vi "MPZ2006固态源.vi"() -> ()   [LabVIEW 2015]
doc: "使用该模板构建用户界面事件处理设计模式。将模板应用于对话框及其它用户界面。用户也可创建并执行VI可按照与用户界面事件相同方式处理的用户定义事件。"
uses:
  <vilib>/Instr/_visa.llb/VISA Configure Serial Port (Instr).vi
panel:
  in  "预备区功率":string
  in  "写入功率控制表":bool caption="按钮1"
  in  "写标定功率检测值":bool caption="按钮1"
  in  "标定参数表":string[][](table)=[["034B", "0412", "04D8", "059F", "0666"], ["149B", "1735", "1A3D", "1D43", "2CCC"], ["15C2", "17AD", "1AE1", "1DE6", "30A3"], ["2851", "2851", "2851", "2851", "2851"], ["2D70", "2D70", "2D70", "2D70", "2D70"]]
  out "功率输出状态":bool
  in  "功率输出":bool
  in  "自动计算参数":bool caption="按钮1"
  in  "读标定功率检测值":bool caption="按钮1"
  in  "偏置2设置 2":dbl max=16383.0 format="%.4f"
  in  "偏置1设置 2":dbl max=16383.0 format="%.4f"
  in  "衰减器2设置 2":dbl max=16383.0 format="%.4f"
  in  "衰减器1设置 2":dbl max=16383.0 format="%.4f"
  out "状态数据":string[](array[string])
  out "串口":bool
  in  "驻波比limit设置":u16=10 min=10 max=99 format="%.0x"
  out "驻波比limit计算":string
  out "驻波比":string
  in  "开始上传":bool caption="按钮1"
  in  "开始下载":bool caption="按钮1"
  out "进度":u8(slide) scale=0.0..100.0
  in  "清空缓冲区":bool caption="按钮1"
  in  "导入模板文件":bool caption="按钮1"
  in  "保存文件":bool caption="按钮1"
  in  "功率控制表":string[][](table)
  in  "偏置2":u16 max=16383 format="%.0x"
  in  "偏置1":u16 max=16383 format="%.0x"
  in  "衰减器2":u16 max=16383 format="%.0x"
  in  "衰减器1":u16 max=16383 format="%.0x"
  in  "复制到数据缓冲区-->":bool caption="按钮1"
  in  "<--复制到控制窗":bool caption="按钮1"
  in  "备注":string
  out "温度limit计算":string
  out "电流limit计算":string
  in  "偏置2设置":u16 max=16383 format="%.0x"
  in  "偏置1设置":u16 max=16383 format="%.0x"
  in  "衰减器2设置":u16 max=16383 format="%.0x"
  in  "衰减器1设置":u16 max=16383 format="%.0x"
  in  "反向功率limit设置":u16 max=4095 format="%.0x"
  in  "正向功率limit设置":u16 max=4095 format="%.0x"
  in  "温度limit设置":u16 max=4095 format="%.0x"
  in  "电流limit设置":u16 max=4095 format="%.0x"
  in  "频率设置":dbl format="%#_6f"
  out "偏置2计算":string
  out "偏置1计算":string
  out "衰减器2计算":string
  out "衰减器1计算":string
  out "反向功率limit计算":string
  out "正向功率limit计算":string
  in  "设置参数":bool caption="按钮1"
  in  "保存数据":bool caption="按钮1"
  out "功率状态":enum16{"OFF", "ON"}(ring)
  out "偏置2 (V)":string
  out "偏置1 (V)":string
  out "衰减器2 (V)":string
  out "衰减器1 (V)":string
  out "驻波比limit":string
  out "反向功率limit (V/W/dBm)":string
  out "正向功率limit (V/W/dBm)":string
  out "温度limit (℃)":string
  out "电流limit（A）":string
  out "反向功率(V/W/dBm)":string
  out "正向功率(V/W/dBm)":string
  out "温度（℃）":string
  out "电流（A）":string
  out "频率（Hz）":string
  out "报警状态":string
  out "功率输出状态":string
  out "SN":string
  out "型号":string
  out "接收的原始数据":string
  in  "波特率":u32(ring)=19200 items=["75"=75, "110"=110, "134"=134, "150"=150, "300"=300, "600"=600, "1200"=1200, "1800"=1800, "2400"=2400, "4800"=4800, "7200"=7200, "9600"=9600, "14400"=14400, "19200"=19200, "28800"=28800, "38400"=38400, "56000"=56000, "57600"=57600, "115200"=115200, "128000"=128000, "230400"=230400]
  in  "串口号":refnum<visa-resource-name>="COM1"
  in  "打开串口":bool caption="按钮1"
  in  "stop":bool caption="停止"
  # "A"
  # "预备区"
  # "℃"
  # "W"
  # "W"
  # "V"
  # "V"
  # "V"
  # "V"
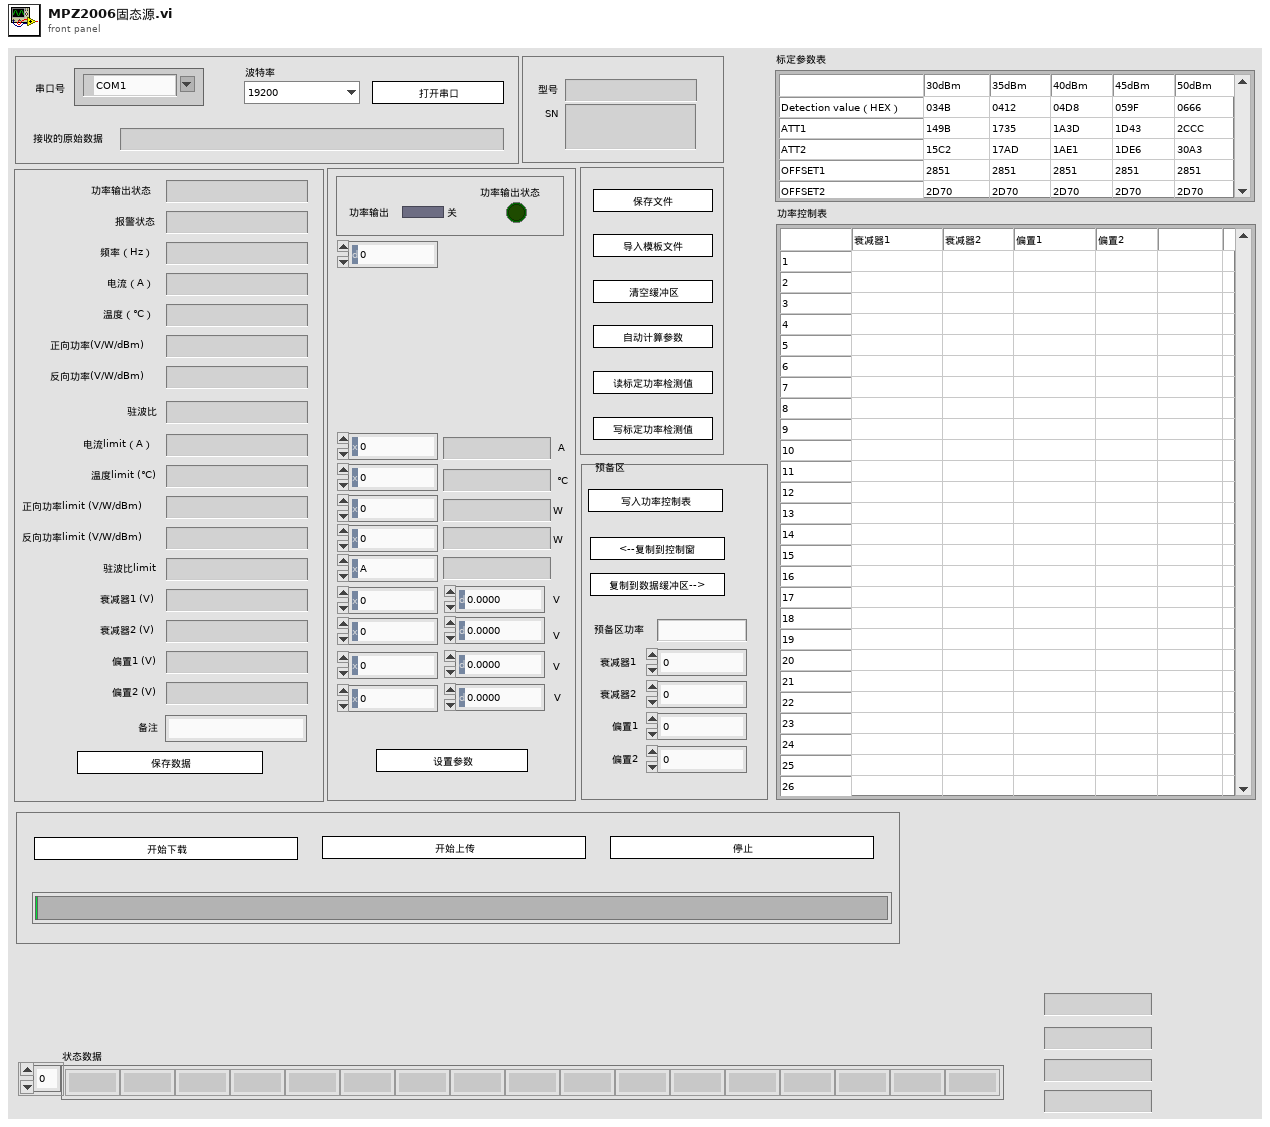
[diagram p1: front panel]
types:
  T1 = cluster{"波特率":u32, "数据比特":u16, "奇偶":enum16{"None", "Odd", "Even", "Mark", "Space"}, "停止位":u16, "流控制":u16}
  T2 = enum8{"Enabled", "Disabled", "Disabled and Grayed Out"}
  T3 = cluster{i16, "频率设置":dbl, "电流limit设置":u16, "温度limit设置":u16, "正向功率limit设置":u16, "反向功率limit设置":u16, "驻波比limit设置":u16, "衰减器1设置":u16, "衰减器2设置":u16, "偏置1设置":u16, "偏置2设置":u16}
  T4 = typedef "LVPoint32TypeDef.ctl" = cluster{"Horizontal":i32, "Vertical":i32}
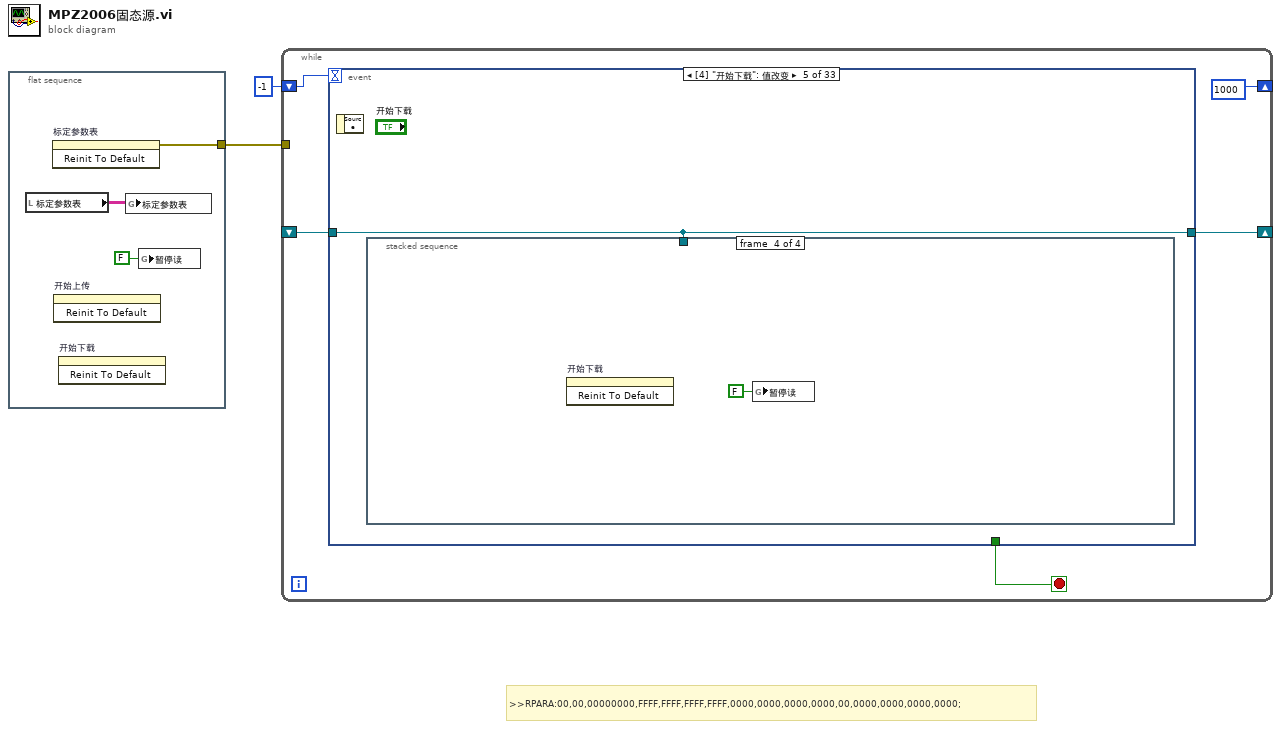
[diagram p0: block diagram]
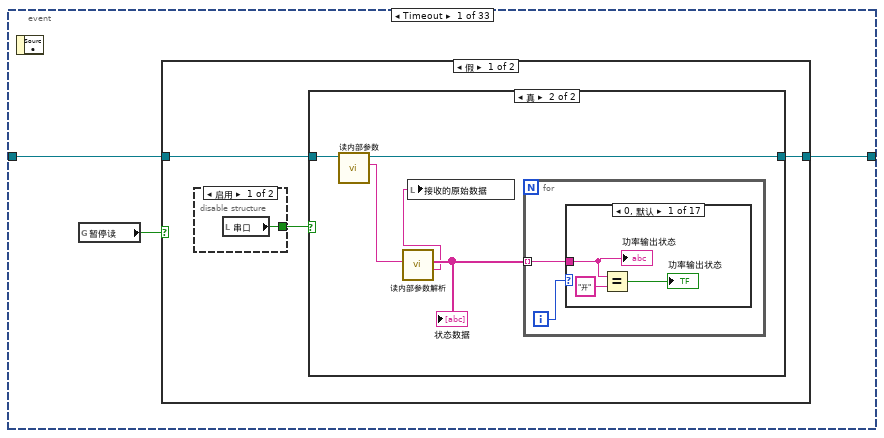
[diagram p2: hidden frame]
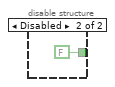
[diagram p3: hidden frame]
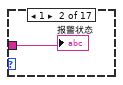
[diagram p5: hidden frame]
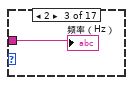
[diagram p6: hidden frame]
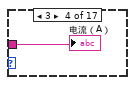
[diagram p7: hidden frame]
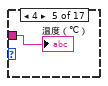
[diagram p8: hidden frame]
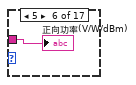
[diagram p9: hidden frame]
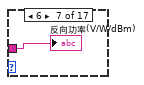
[diagram p10: hidden frame]
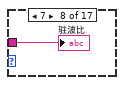
[diagram p11: hidden frame]
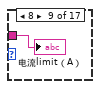
[diagram p12: hidden frame]
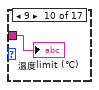
[diagram p13: hidden frame]
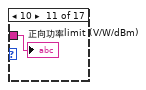
[diagram p14: hidden frame]
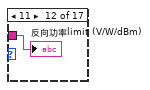
[diagram p15: hidden frame]
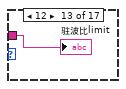
[diagram p16: hidden frame]
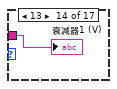
[diagram p17: hidden frame]
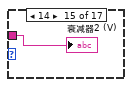
[diagram p18: hidden frame]
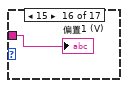
[diagram p19: hidden frame]
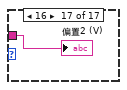
[diagram p20: hidden frame]
diagram:
  # ">>RPARA:00,00,00000000,FFFF,FFFF,FFFF,FFFF,0000,0000,0000,0000,00,0000,0000,0000,0000;"
  n1 = flat-sequence {
    tunnel: [w5] -> w1
    frame #0 {
      n2 = local read "标定参数表"() -> (w4:string[][])
      n3 = invoke on="标定参数表" class="Tbl (严格)" method="Reinit To Default"() -> (error out=w5:errorcluster)  [unwired: 3 in, 2 out]
      n4 = invoke on="开始上传" class="Bool (严格)" method="Reinit To Default"() -> ()  [unwired: 3 in, 3 out]
      n5 = invoke on="开始下载" class="Bool (严格)" method="Reinit To Default"() -> ()  [unwired: 3 in, 3 out]
      n6 = global write "Globle.vi" "标定参数表"(w4) -> ()
      n7 = global write "Globle.vi" "暂停读"(FALSE ("暂停读")) -> ()
    }
  }
  n8 = while {
    shift-right: [w9] -> _
    shift-left: _ -> [w7]
    shift-right: [1000] -> _
    shift-left: -1 -> [w8]
    tunnel: w1 -> [_]
    stop <- w10 stop-if-true
    n9 = event shown="[4] \"开始下载\": 值改变" {
      selector: _ -> [_ _ _ _ _ _ _ _ _ _ _ _ _ _ _ _ _ _ _ _ _ _ _ _ _ _ _ _ _ _ _ _ _]
      dyn-events: _ -> [_ _ _ _ _ _ _ _ _ _ _ _ _ _ _ _ _ _ _ _ _ _ _ _ _ _ _ _ _ _ _ _ _]
      timeout: w8 -> [_ _ _ _ _ _ _ _ _ _ _ _ _ _ _ _ _ _ _ _ _ _ _ _ _ _ _ _ _ _ _ _ _]
      tunnel: [_ _ _ _ _ _ _ _ _ _ _ _ _ _ _ _ _ _ _ _ _ _ _ _ _ _ _ _ _ _ _ "stop" TRUE] -> w10
      tunnel: [w12 w51 w79 w105 w106 w130 w155 w163 w169 w177 w185 w192 w200 w208 w216 w228 w234 w240 w246 w248 w253 w254 w266 w280 w283 w287 w294 w299 w303 w317 w318 _ _] -> w9
      tunnel: w7 -> [w13 w49 w79 w105 w106 w130 w155 w163 w169 w177 w185 w192 w200 w208 w216 w228 w234 w240 w246 w248 w253 w254 w266 w280 w283 w287 w294 w299 w303 w317 w318 w323 w326]
      event Timeout {
        n10 = event-data() -> ()  [unwired: 1 in, 1 out]
        n11 = global read "Globle.vi" "暂停读"() -> (w11:bool)
        n12 = case shown="假" w11 {
          tunnel: w13 -> [w16 w46]
          tunnel: [w15 w46] -> w12
          frame False {
            n13 = disable-structure shown="启用" {
              disable-tunnel: [w17 FALSE ("串口")] -> w14
              frame Enabled {
                n14 = local read "串口"() -> (w17:bool)
              }
              frame Disabled {
              }
            }
            n15 = case shown="真" w14 {
              tunnel: w16 -> [w19 w24]
              tunnel: [w19 w23] -> w15
              frame False {
              }
              frame True {
                n16 = call "读内部参数.vi"("VISA资源名称"=w24) -> ("响应"=w21:string, "VISA资源名称 2"=w23:refnum<visa-resource-name>)  [unwired: 9 in]
                n17 = call "读内部参数解析.vi"("响应"=w21) -> ("消息"=w20:string, "读内部参数"=w22:string[])  [unwired: 9 in]
                "状态数据" <- w22
                n18 = local write "接收的原始数据"(w20) -> ()
                n19 = for {
                  tunnel: w22 -> [w25] mode=indexing
                  i -> [w26]
                  n20 = case shown="0, 默认" w26 {
                    tunnel: w25 -> [w29 w30 w31 w32 w33 w34 w35 w36 w37 w38 w39 w40 w41 w42 w43 w44 w45]
                    frame 0, Default {
                      n21 = Equal?(x=w29, y="开") -> (x = y?=→"功率输出状态":bool)
                      "功率输出状态" <- w29
                    }
                    frame 1 {
                      "报警状态" <- w30
                    }
                    frame 2 {
                      "频率（Hz）" <- w31
                    }
                    frame 3 {
                      "电流（A）" <- w32
                    }
                    frame 4 {
                      "温度（℃）" <- w33
                    }
                    frame 5 {
                      "正向功率(V/W/dBm)" <- w34
                    }
                    frame 6 {
                      "反向功率(V/W/dBm)" <- w35
                    }
                    frame 7 {
                      "驻波比" <- w36
                    }
                    frame 8 {
                      "电流limit（A）" <- w37
                    }
                    frame 9 {
                      "温度limit (℃)" <- w38
                    }
                    frame 10 {
                      "正向功率limit (V/W/dBm)" <- w39
                    }
                    frame 11 {
                      "反向功率limit (V/W/dBm)" <- w40
                    }
                    frame 12 {
                      "驻波比limit" <- w41
                    }
                    frame 13 {
                      "衰减器1 (V)" <- w42
                    }
                    frame 14 {
                      "衰减器2 (V)" <- w43
                    }
                    frame 15 {
                      "偏置1 (V)" <- w44
                    }
                    frame 16 {
                      "偏置2 (V)" <- w45
                    }
                  }
                }
              }
            }
          }
          frame True {
          }
        }
      }
      event "打开串口": Value Change {
        n22 = event-data() -> ("NewVal"=w50:bool)  [unwired: 1 in]
        n23 = case shown="真" w50 {
          tunnel: [_ w56] -> w51
          tunnel: w49 -> [w53 _]
          tunnel: [FALSE w54] -> w47
          frame False {
            n24 = VISA Close(VISA resource name=w53) -> ()  [unwired: 1 in, 1 out]
          }
          frame True {
            n25 = Bundle By Name(cluster=T1 {"波特率"=9600, "数据比特"=8, "奇偶"=enum."None", "停止位"=10, "流控制"=0} ("串口设置"), "波特率"="波特率") -> (w59:T1)
            n26 = Unbundle By Name(w59) -> ("波特率"=w63:u32, "数据比特"=w64:u16, "奇偶"=w65:enum16{"None", "Odd", "Even", "Mark", "Space"}, "停止位"=w66:u16, "流控制"=w67:u16)
            n27 = call-poly "VISA Configure Serial Port"("VISA resource name"="串口号", "baud rate (9600)"=w63, "data bits (8)"=w64, "parity (0:none)"=w65, "stop bits (10: 1 bit)"=w66, "flow control (0:none)"=w67) -> ("VISA resource name out"=w57:refnum<visa-resource-name>, "error out"=w58:errorcluster)  [unwired: 3 in, 5 out]
            n28 = case shown="无错误" w58 {
              tunnel: w57 -> [w74 w78]
              tunnel: [w73 w78] -> w56
              tunnel: [TRUE FALSE] -> w54
              tunnel: [T2."Enabled" ("禁用") T2."Disabled and Grayed Out" ("禁用")] -> w55
              frame No Error {
                n29 = call "查询设备信息.vi"("VISA资源名称"=w74) -> ("响应"=w70:string, "VISA资源名称 2"=w73:refnum<visa-resource-name>)  [unwired: 8 in, 1 out]
                "接收的原始数据" <- w70
                n30 = call "查询设备信息解析.vi"("响应"=w70) -> ("SN"=→"SN":string, "型号"=→"型号":string)  [unwired: 9 in]
              }
              frame Error {
                n31 = local write "接收的原始数据"("串口连接错误。" ("消息")) -> ()
              }
            }
            n32 = property on="设置参数" class="Bool"("DisabledEnum"=w55) -> ()  [unwired: 2 in, 2 out]
          }
        }
        "串口" <- w47
        n33 = local write "进度"(0) -> ()
      }
      event "设置参数": Value Change {
        n34 = event-data() -> ()  [unwired: 1 in, 1 out]
        n35 = local read "正向功率limit设置"() -> (w90:u16)
        n36 = local read "反向功率limit设置"() -> (w89:u16)
        n37 = local read "驻波比limit设置"() -> (w88:u16)
        n38 = local read "电流limit设置"() -> (w92:u16)
        n39 = local read "温度limit设置"() -> (w91:u16)
        n40 = local read "衰减器1设置"() -> (w87:u16)
        n41 = local read "衰减器2设置"() -> (w86:u16)
        n42 = local read "偏置1设置"() -> (w85:u16)
        n43 = local read "偏置2设置"() -> (w84:u16)
        n44 = Boolean To (0,1)(Boolean="功率输出") -> (0, 1=w81:i16)
        "功率状态" <- w81
        n45 = Bundle(w81, "频率设置"="频率设置", "电流limit设置"=w92, "温度limit设置"=w91, "正向功率limit设置"=w90, "反向功率limit设置"=w89, "驻波比limit设置"=w88, "衰减器1设置"=w87, "衰减器2设置"=w86, "偏置1设置"=w85, "偏置2设置"=w84) -> (w83:T3)  [unwired: 1 in]
        n46 = call "参数簇转换字符串.vi"("设置参数簇"=w83) -> ("输入参数"=w82:string)  [unwired: 10 in]
        n47 = stacked-sequence {
          tunnel: w82 -> [_ _ w98 _]
          tunnel: w79 -> [_ _ w97 _]
          frame #0 {
            n48 = global write "Globle.vi" "暂停读"(TRUE ("暂停读")) -> ()
          }
          frame #1 {
            n49 = Wait (ms)(milliseconds to wait=u32 1000 ("等待时间（毫秒）")) -> ()  [unwired: 1 out]
          }
          frame #2 {
            n50 = call "写内部参数.vi"("参数"=w98, "VISA资源名称"=w97) -> ("响应"=w96:string)  [unwired: 8 in, 1 out]
            n51 = local write "接收的原始数据"(w96) -> ()
            n52 = call "写内部参数解析.vi"("响应"=w96) -> ()  [unwired: 10 in, 1 out]
          }
          frame #3 {
            n53 = global write "Globle.vi" "暂停读"(FALSE ("暂停读")) -> ()
          }
        }
      }
      event "保存数据": Value Change {
        n54 = event-data() -> ()  [unwired: 1 in, 1 out]
        n55 = control-ref of="该应用程序"() -> (w100:refnum<vi>)
        n56 = local read "状态数据"() -> (w104:string[])
        n57 = local read "型号"() -> (w103:string)
        n58 = local read "SN"() -> (w102:string)
        n59 = call "保存数据.vi"("备注"="备注", "状态数据"=w104, "应用程序输入"=w100, "SN"=w102, "型号"=w103) -> ()  [unwired: 7 in]
      }
      event "开始下载": Value Change {
        n60 = event-data() -> ()  [unwired: 1 in, 1 out]
        n61 = stacked-sequence {
          tunnel: w106 -> [_ _ w113 _]
          frame #0 {
            n62 = global write "Globle.vi" "暂停读"(TRUE ("暂停读")) -> ()
          }
          frame #1 {
            n63 = Wait (ms)(milliseconds to wait=u32 1000 ("等待时间（毫秒）")) -> ()  [unwired: 1 out]
          }
          frame #2 {
            n64 = call "文件对话框"("prompt"="选择模板", "pattern (all files)"="*.xlsx") -> ("selected path"=w111:path, "cancelled"=w110:bool)  [unwired: 10 in, 2 out]
            n65 = case shown="真" w110 {
              tunnel: w113 -> [w118 _]
              tunnel: w111 -> [w115 _]
              frame False {
                n66 = flat-sequence {
                  tunnel: [w121] -> w116
                  tunnel: w115 -> [w120]
                  tunnel: [w120] -> w114
                  frame #0 {
                    w121 = u8 0 ("进度")
                    n67 = global write "Globle.vi" "进度条"(FALSE ("进度条")) -> ()
                    n68 = global write "Globle.vi" "行号"(w121) -> ()
                    n69 = local write "进度"(w121) -> ()
                  }
                }
                n70 = while {
                  tunnel: w116 -> [_]
                  stop <- w126 stop-if-true
                  n71 = global read "Globle.vi" "行号"() -> (w122:u32)
                  "进度" <- w122
                  n72 = Wait (ms)(milliseconds to wait=u32 500 ("等待时间（毫秒）")) -> ()  [unwired: 1 out]
                  n73 = global read "Globle.vi" "进度条"() -> (w125:bool)
                  n74 = Equal?(x=101, y=w122) -> (x = y?=w123:bool)
                  n75 = Or(x=w123, y=w125) -> (x .or. y?=w126:bool)
                  n76 = case shown="真" w123 {
                    frame False {
                    }
                    frame True {
                      n77 = One Button Dialog(message="下载完成。") -> ()  [unwired: 1 in, 1 out]
                    }
                  }
                }
                n78 = call "写文件main.vi"("下载路径"=w114, "VISA资源名称"=w118) -> ("消息"=w117:string)  [unwired: 8 in, 1 out]
                n79 = local write "接收的原始数据"(w117) -> ()
              }
              frame True {
                n80 = invoke on="开始下载" class="Bool (严格)" method="Reinit To Default"() -> ()  [unwired: 3 in, 3 out]
              }
            }
          }
          frame #3 {
            n81 = invoke on="开始下载" class="Bool (严格)" method="Reinit To Default"() -> ()  [unwired: 3 in, 3 out]
            n82 = global write "Globle.vi" "暂停读"(FALSE ("暂停读")) -> ()
          }
        }
      }
      event "开始上传": Value Change {
        n83 = event-data() -> ()  [unwired: 1 in, 1 out]
        n84 = stacked-sequence {
          tunnel: w130 -> [_ _ w137 _]
          frame #0 {
            n85 = global write "Globle.vi" "暂停读"(TRUE ("暂停读")) -> ()
          }
          frame #1 {
            n86 = Wait (ms)(milliseconds to wait=u32 1000 ("等待时间（毫秒）")) -> ()  [unwired: 1 out]
          }
          frame #2 {
            n87 = call "文件对话框2"("prompt"="输入文件名", "pattern (all files)"="*.xlsx") -> ("selected path"=w134:path, "cancelled"=w135:bool)  [unwired: 10 in, 2 out]
            n88 = case shown="真" w135 {
              tunnel: w137 -> [w143 _]
              tunnel: w134 -> [w139 _]
              frame False {
                n89 = flat-sequence {
                  tunnel: [w146] -> w141
                  tunnel: w139 -> [w145]
                  tunnel: [w145] -> w138
                  frame #0 {
                    w146 = u8 0 ("进度")
                    n90 = global write "Globle.vi" "进度条"(FALSE ("进度条")) -> ()
                    n91 = global write "Globle.vi" "行号"(w146) -> ()
                    n92 = local write "进度"(w146) -> ()
                  }
                }
                n93 = control-ref of="该应用程序"() -> (w140:refnum<vi>)
                n94 = while {
                  tunnel: w141 -> [_]
                  stop <- w151 stop-if-true
                  n95 = global read "Globle.vi" "行号"() -> (w147:u32)
                  n96 = Wait (ms)(milliseconds to wait=u32 500 ("等待时间（毫秒）")) -> ()  [unwired: 1 out]
                  n97 = global read "Globle.vi" "进度条"() -> (w150:bool)
                  n98 = local write "进度"(w147) -> ()
                  n99 = Equal?(x=100, y=w147) -> (x = y?=w148:bool)
                  n100 = Or(x=w148, y=w150) -> (x .or. y?=w151:bool)
                  n101 = case shown="真" w148 {
                    frame False {
                    }
                    frame True {
                      n102 = One Button Dialog(message="上传完成。") -> ()  [unwired: 1 in, 1 out]
                    }
                  }
                }
                n103 = call "读文件main.vi"("保存路径"=w138, "应用程序输入"=w140, "VISA资源名称"=w143) -> ("消息"=w142:string)  [unwired: 6 in, 2 out]
                n104 = local write "接收的原始数据"(w142) -> ()
              }
              frame True {
                n105 = invoke on="开始上传" class="Bool (严格)" method="Reinit To Default"() -> ()  [unwired: 3 in, 3 out]
              }
            }
          }
          frame #3 {
            n106 = invoke on="开始上传" class="Bool (严格)" method="Reinit To Default"() -> ()  [unwired: 3 in, 3 out]
            n107 = global write "Globle.vi" "暂停读"(FALSE ("暂停读")) -> ()
          }
        }
      }
      event "电流limit设置": Value Change {
        n108 = event-data() -> ()  [unwired: 1 in, 1 out]
        n109 = Multiply(x="电流limit设置", y=0.0008056640625) -> (x*y=w160:dbl)
        n110 = Divide(x=w160, y=0.05) -> (x/y=w158:dbl)
        n111 = Number To Fractional String(number=w158, precision (6)=i16 5 ("精度(6)")) -> (F-format string=→"电流limit计算":string)  [unwired: 2 in]
      }
      event "温度limit设置": Value Change {
        n112 = event-data() -> ()  [unwired: 1 in, 1 out]
        n113 = Divide(x="温度limit设置", y=10.0) -> (x/y=w166:dbl)
        n114 = Number To Fractional String(number=w166, precision (6)=i16 1 ("精度(6)")) -> (F-format string=→"温度limit计算":string)  [unwired: 2 in]
      }
      event "正向功率limit设置": Value Change {
        n115 = event-data() -> ()  [unwired: 1 in, 1 out]
        n116 = Divide(x="正向功率limit设置", y=4095.0) -> (x/y=w174:dbl)
        n117 = Multiply(x=w174, y=3.3) -> (x*y=w172:dbl)
        n118 = Number To Fractional String(number=w172, precision (6)=i16 5 ("精度(6)")) -> (F-format string=→"正向功率limit计算":string)  [unwired: 2 in]
      }
      event "反向功率limit设置": Value Change {
        n119 = event-data() -> ()  [unwired: 1 in, 1 out]
        n120 = Divide(x="反向功率limit设置", y=4095.0) -> (x/y=w183:dbl)
        n121 = Multiply(x=w183, y=3.3) -> (x*y=w181:dbl)
        n122 = Number To Fractional String(number=w181, precision (6)=i16 5 ("精度(6)")) -> (F-format string=→"反向功率limit计算":string)  [unwired: 2 in]
      }
      event "驻波比limit设置": Value Change {
        n123 = event-data() -> ()  [unwired: 1 in, 1 out]
        n124 = Divide(x="驻波比limit设置", y=10.0) -> (x/y=w186:dbl)
        n125 = Number To Fractional String(number=w186, precision (6)=i16 1 ("精度(6)")) -> (F-format string=→"驻波比limit计算":string)  [unwired: 2 in]
      }
      event "衰减器1设置": Value Change {
        n126 = event-data() -> ()  [unwired: 1 in, 1 out]
        n127 = local read "衰减器1设置"() -> (w198:u16)
        n128 = Divide(x=w198, y=16383.0) -> (x/y=w196:dbl)
        n129 = Multiply(x=w196, y=5.0) -> (x*y=w191:dbl)
        n130 = Number To Fractional String(number=w191, precision (6)=i16 5 ("精度(6)")) -> (F-format string=→"衰减器1计算":string)  [unwired: 2 in]
        n131 = local write "衰减器1设置 2"(w191) -> ()
      }
      event "衰减器2设置": Value Change {
        n132 = event-data() -> ()  [unwired: 1 in, 1 out]
        n133 = local read "衰减器2设置"() -> (w203:u16)
        n134 = Divide(x=w203, y=16383.0) -> (x/y=w202:dbl)
        n135 = Multiply(x=w202, y=5.0) -> (x*y=w199:dbl)
        n136 = Number To Fractional String(number=w199, precision (6)=i16 5 ("精度(6)")) -> (F-format string=→"衰减器2计算":string)  [unwired: 2 in]
        n137 = local write "衰减器2设置 2"(w199) -> ()
      }
      event "偏置1设置": Value Change {
        n138 = event-data() -> ()  [unwired: 1 in, 1 out]
        n139 = local read "偏置1设置"() -> (w214:u16)
        n140 = Divide(x=w214, y=16383.0) -> (x/y=w210:dbl)
        n141 = Multiply(x=w210, y=5.0) -> (x*y=w207:dbl)
        n142 = Number To Fractional String(number=w207, precision (6)=i16 5 ("精度(6)")) -> (F-format string=→"偏置1计算":string)  [unwired: 2 in]
        n143 = local write "偏置1设置 2"(w207) -> ()
      }
      event "偏置2设置": Value Change {
        n144 = event-data() -> ()  [unwired: 1 in, 1 out]
        n145 = local read "偏置2设置"() -> (w218:u16)
        n146 = Divide(x=w218, y=16383.0) -> (x/y=w220:dbl)
        n147 = Multiply(x=w220, y=5.0) -> (x*y=w215:dbl)
        n148 = Number To Fractional String(number=w215, precision (6)=i16 5 ("精度(6)")) -> (F-format string=→"偏置2计算":string)  [unwired: 2 in]
        n149 = local write "偏置2设置 2"(w215) -> ()
      }
      event "衰减器1设置 2": Value Change {
        n150 = event-data() -> ()  [unwired: 1 in, 1 out]
        n151 = Divide(x="衰减器1设置 2", y=5.0) -> (x/y=w225:dbl)
        n152 = Multiply(x=w225, y=16383.0) -> (x*y=w223:dbl)
        n153 = local write "衰减器1设置"(w223) -> ()
      }
      event "衰减器2设置 2": Value Change {
        n154 = event-data() -> ()  [unwired: 1 in, 1 out]
        n155 = Divide(x="衰减器2设置 2", y=5.0) -> (x/y=w232:dbl)
        n156 = Multiply(x=w232, y=16383.0) -> (x*y=w230:dbl)
        n157 = local write "衰减器2设置"(w230) -> ()
      }
      event "偏置1设置 2": Value Change {
        n158 = event-data() -> ()  [unwired: 1 in, 1 out]
        n159 = Divide(x="偏置1设置 2", y=5.0) -> (x/y=w238:dbl)
        n160 = Multiply(x=w238, y=16383.0) -> (x*y=w236:dbl)
        n161 = local write "偏置1设置"(w236) -> ()
      }
      event "偏置2设置 2": Value Change {
        n162 = event-data() -> ()  [unwired: 1 in, 1 out]
        n163 = Divide(x="偏置2设置 2", y=5.0) -> (x/y=w244:dbl)
        n164 = Multiply(x=w244, y=16383.0) -> (x*y=w242:dbl)
        n165 = local write "偏置2设置"(w242) -> ()
      }
      event "标定参数表": Value Change {
        n166 = event-data() -> ()  [unwired: 1 in, 1 out]
        n167 = local read "标定参数表"() -> (w247:string[][])
        n168 = global write "Globle.vi" "标定参数表"(w247) -> ()
      }
      event "保存文件": Value Change {
        n169 = event-data() -> ()  [unwired: 1 in, 1 out]
        n170 = local read "SN"() -> (w249:string)
        n171 = control-ref of="该应用程序"() -> (w252:refnum<vi>)
        n172 = control-ref of="标定参数表"() -> (w251:refnum<vi>)
        n173 = control-ref of="功率控制表"() -> (w250:refnum<vi>)
        n174 = call "保存功率控制表和标定参数表.vi"("SN"=w249, "功率控制表"=w250, "标定参数表"=w251, "该应用程序"=w252) -> ()  [unwired: 8 in]
      }
      event "读标定功率检测值": Value Change {
        n175 = event-data() -> ()  [unwired: 1 in, 1 out]
        n176 = stacked-sequence {
          tunnel: w254 -> [_ _ w263 _ _]
          frame #0 {
            n177 = global write "Globle.vi" "暂停读"(TRUE ("暂停读")) -> ()
          }
          frame #1 {
            n178 = Wait (ms)(milliseconds to wait=u32 1000 ("等待时间（毫秒）")) -> ()  [unwired: 1 out]
          }
          frame #2 {
            n179 = call "读标定功率检测值.vi"("VISA资源名称"=w263) -> ("响应"=w262:string)  [unwired: 9 in, 1 out]
            n180 = call "读标定功率检测值解析.vi"("响应"=w262) -> ("消息"=w261:string, "读标定功率检测值"=w260:string[])  [unwired: 9 in]
            n181 = local write "接收的原始数据"(w261) -> ()
            n182 = Replace Array Subset(array="标定参数表", new element=w260, index (row)=0 ("索引 (行)")) -> (w257:string[][])  [unwired: 1 in]
            n183 = local write "标定参数表"(w257) -> ()
            n184 = global write "Globle.vi" "标定参数表"(w257) -> ()
          }
          frame #3 {
            n185 = global write "Globle.vi" "暂停读"(FALSE ("暂停读")) -> ()
          }
          frame #4 {
            n186 = One Button Dialog(message="读标定功率检测值完成。" ("消息")) -> ()  [unwired: 1 in, 1 out]
          }
        }
      }
      event "写标定功率检测值": Value Change {
        n187 = event-data() -> ()  [unwired: 1 in, 1 out]
        n188 = stacked-sequence {
          tunnel: w266 -> [_ _ w275 _ _]
          frame #0 {
            n189 = global write "Globle.vi" "暂停读"(TRUE ("暂停读")) -> ()
          }
          frame #1 {
            n190 = Wait (ms)(milliseconds to wait=u32 1000 ("等待时间（毫秒）")) -> ()  [unwired: 1 out]
          }
          frame #2 {
            n191 = local read "标定参数表"() -> (w273:string[][])
            n192 = Index Array(array=w273, index (row)=0 ("禁用的索引 (列)")) -> (element=w271:string[])  [unwired: 1 in]
            n193 = call <userlib>:"1D Array to String__ogtk.vi"("delimiter (Tab)"=",", "Array of Strings"=w271) -> ("delimited string"=w270:string)  [unwired: 9 in]
            n194 = call "写标定功率检测值.vi"("参数"=w270, "VISA资源名称"=w275) -> ("响应"=w269:string)  [unwired: 8 in, 1 out]
            n195 = call "写标定功率检测值解析.vi"("响应"=w269) -> ()  [unwired: 11 in]
          }
          frame #3 {
            n196 = global write "Globle.vi" "暂停读"(FALSE ("暂停读")) -> ()
          }
          frame #4 {
            n197 = One Button Dialog(message="写标定功率检测值完成。" ("消息")) -> ()  [unwired: 1 in, 1 out]
          }
        }
      }
      event "导入模板文件": Value Change {
        n198 = event-data() -> ()  [unwired: 1 in, 1 out]
        n199 = control-ref of="标定参数表"() -> (w279:refnum<vi>)
        n200 = control-ref of="功率控制表"() -> (w278:refnum<vi>)
        n201 = call "导入模板文件.vi"("功率控制表"=w278, "标定参数表"=w279) -> ()  [unwired: 10 in]
      }
      event "清空缓冲区": Value Change {
        n202 = event-data() -> ()  [unwired: 1 in, 1 out]
        n203 = control-ref of="功率控制表"() -> (w282:refnum<vi>)
        n204 = property class="Tbl (严格)"(reference=w282, "Value"=string[][] [] ("值")) -> ()  [unwired: 1 in, 2 out]
      }
      event "自动计算参数": Value Change {
        n205 = event-data() -> ()  [unwired: 1 in, 1 out]
        n206 = control-ref of="该应用程序"() -> (w286:refnum<vi>)
        n207 = control-ref of="标定参数表"() -> (w285:refnum<vi>)
        n208 = control-ref of="功率控制表"() -> (w284:refnum<vi>)
        n209 = call "自动计算参数.vi"("功率控制表"=w284, "标定参数表"=w285, "应用程序输入"=w286) -> ()  [unwired: 9 in]
      }
      event "写入功率控制表": Value Change {
        n210 = event-data() -> ()  [unwired: 1 in, 1 out]
        n211 = local read "衰减器1"() -> (w292:u16)
        n212 = local read "衰减器2"() -> (w291:u16)
        n213 = local read "偏置1"() -> (w290:u16)
        n214 = local read "偏置2"() -> (w289:u16)
        n215 = control-ref of="功率控制表"() -> (w293:refnum<vi>)
        n216 = call "写入功率控制表.vi"("预备区功率"="预备区功率", "Table输入"=w293, "偏置2"=w289, "偏置1"=w290, "衰减器2"=w291, "衰减器1"=w292) -> ()  [unwired: 6 in]
      }
      event "功率控制表": Shortcut Menu Activation? {
        n217 = event-data() -> ("MenuRef"=w295:refnum<k9>)  [unwired: 1 in]
        n218 = Delete Menu Items(9:w295) -> (0:w297:errorcluster, 3:w298:refnum<k9>)  [unwired: 3 in]
        n219 = Insert Menu Items(6:w297, 7:string[] ["拷贝到预备区", "绘制曲线"] ("L10n_item tags 1"), 9:w298) -> ()  [unwired: 3 in, 3 out]
        n220 = event-data() -> ()  [unwired: 2 in, 1 out]
      }
      event "功率控制表": Shortcut Menu Selection (User) {
        n221 = event-data() -> ("ItemTag"=w302:string, "CtlRef"=w300:refnum<vi>, "Coords"=w301:T4)  [unwired: 1 in]
        n222 = case shown="\"拷贝到预备区\", 默认" w302 {
          tunnel: w301 -> [w311 _]
          tunnel: w300 -> [w310 _]
          frame "拷贝到预备区", Default {
            n223 = call "拷贝到预备区.vi"("Coords"=w311, "CtlRef"=w310) -> ("预备区功率"=w309:string, "衰减/偏置"=w308:u32[])  [unwired: 8 in]
            n224 = local write "预备区功率"(w309) -> ()
            n225 = Index Array(array=w308) -> (element #1=w307:u32, element #2=w306:u32, element #3=w305:u32, element #4=w304:u32)  [unwired: 4 in]
            n226 = local write "衰减器1"(w307) -> ()
            n227 = local write "衰减器2"(w306) -> ()
            n228 = local write "偏置1"(w305) -> ()
            n229 = local write "偏置2"(w304) -> ()
          }
          frame "绘制曲线" {
            n230 = control-ref of="功率控制表"() -> (w312:refnum<vi>)
            n231 = call "功率电压图.vi"("功率控制表"=w312) -> ()  [unwired: 11 in]
          }
        }
      }
      event "<--复制到控制窗": Value Change {
        n232 = event-data() -> ()  [unwired: 1 in, 1 out]
        n233 = property on="衰减器1设置" class="DigNum (严格)"("Val(Sgnl)"="衰减器1") -> ()  [unwired: 2 in, 2 out]
        n234 = property on="衰减器2设置" class="DigNum (严格)"("Val(Sgnl)"="衰减器2") -> ()  [unwired: 2 in, 2 out]
        n235 = property on="偏置1设置" class="DigNum (严格)"("Val(Sgnl)"="偏置1") -> ()  [unwired: 2 in, 2 out]
        n236 = property on="偏置2设置" class="DigNum (严格)"("Val(Sgnl)"="偏置2") -> ()  [unwired: 2 in, 2 out]
      }
      event "复制到数据缓冲区-->": Value Change {
        n237 = event-data() -> ()  [unwired: 1 in, 1 out]
        n238 = local write "偏置2"("偏置2设置") -> ()
        n239 = local write "偏置1"("偏置1设置") -> ()
        n240 = local write "衰减器1"("衰减器1设置") -> ()
        n241 = local write "衰减器2"("衰减器2设置") -> ()
      }
      event "stop": Value Change {
        n242 = event-data() -> ()  [unwired: 1 in, 1 out]
        n243 = VISA Close(VISA resource name=w323) -> ()  [unwired: 1 in, 1 out]
      }
      event Application Instance Close {
        n244 = event-data() -> ()  [unwired: 1 in, 1 out]
        n245 = VISA Close(VISA resource name=w326) -> ()  [unwired: 1 in, 1 out]
      }
    }
  }
